vi "delay time (SubVI).vi"(2 "Time Setpoint (s)":dbl=10.0, 3 "START/RESET TIMER":bool) -> (0 "Time (s)":dbl, 1 "Time Elapsed":bool)   [LabVIEW 2012]
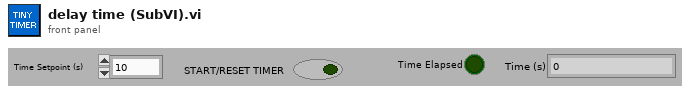
[diagram p1: front panel]
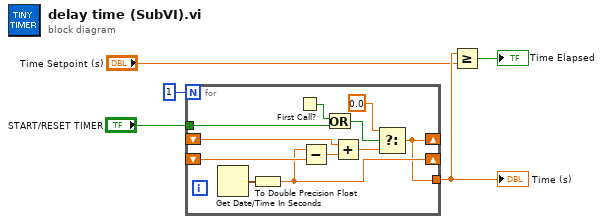
[diagram p0: block diagram]
diagram:
  n1 = for "Timer" {
    N: 1 -> [_]
    shift-right: [w12] -> _
    shift-left: _ -> [w16]
    shift-right: [w13] -> _
    shift-left: _ -> [w15]
    tunnel: [w12] -> w2
    tunnel: "START/RESET TIMER" -> [w6]
    n2 = Get Date/Time In Seconds() -> (seconds since 1Jan1904=w14:timestamp)
    n3 = To Double Precision Float(number=w14) -> (double precision float=w13:dbl)
    n4 = First Call?() -> (First Call?: T/F=w7:bool)
    n5 = Subtract(x=w13, y=w15) -> (x-y=w11:dbl)
    n6 = Or(x=w7, y=w6) -> (x .or. y?=w8:bool)
    n7 = Add(x=w16, y=w11) -> (x+y=w10:dbl)
    n8 = Select(t=0.0, s=w8, f=w10) -> (s? t:f=w12:dbl)
  }
  "Time (s)" <- w2
  n9 = Greater Or Equal?(x=w2, y="Time Setpoint (s)") -> (x >= y?=→"Time Elapsed":bool)
